vi "Example_SOM.vi"() -> ()   [LabVIEW 2009]
uses:
  <vilib>/addons/Machine Learning/Unsupervised Learning/ml_SOM_structure.ctl
  <vilib>/addons/Machine Learning/Unsupervised Learning/ml_SOM_Kohonen Para.ctl
  <vilib>/Utility/miscctls.llb/LV3DPointTypeDef.ctl
  <vilib>/addons/Machine Learning/Visualization/Plot SOM (3D).vi
  <vilib>/addons/Machine Learning/Utilities/Riffle (matrix).vi
  <vilib>/addons/Machine Learning/NILabs_MLT.lvlib
panel:
  in  "Data set":T1(ring)
  in  "Stopping criteria":cluster{"tolarence":dbl, "max iterations":i32}={"tolarence"=1e-05, "max iterations"=50}
  in  "Parameters":T2={"d0"=5.0, "k_d"=5000.0, "miu0"=0.5, "k_miu"=500.0}
  in  "Lattice structure":T3={"row"=7, "col"=7, "lattice type"=enum."rectangular"}
  in  "# of samples":i32=1024
  out "SOM in the data space":refnum<vi>(3d-picture)
  # "Introduction:\nSelf-Organizing Map (SOM) is used to learn four data sets which have different structures."
  # "Data samples (red dots)\nNeurons (green dots) are conneted according to SOM lattice structure."
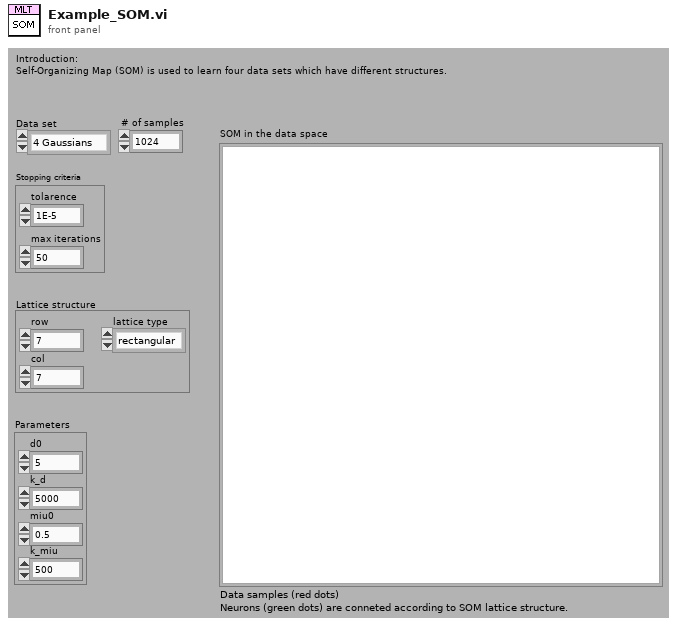
[diagram p1: front panel]
types:
  T1 = enum16{"4 Gaussians ", "uniform", "3 balls", "hemisphere"}
  T2 = typedef "NILabs_MLT.lvlib/ml_SOM_Kohonen Para.ctl" = cluster{"d0":dbl, "k_d":dbl, "miu0":dbl, "k_miu":dbl}
  T3 = typedef "NILabs_MLT.lvlib/ml_SOM_structure.ctl" = cluster{"row":i32, "col":i32, "lattice type":enum16{"rectangular", "hexagonal"}}
  T4 = typedef "LV3DPointTypeDef.ctl" = cluster{"X":sgl, "Y":sgl, "Z":sgl}
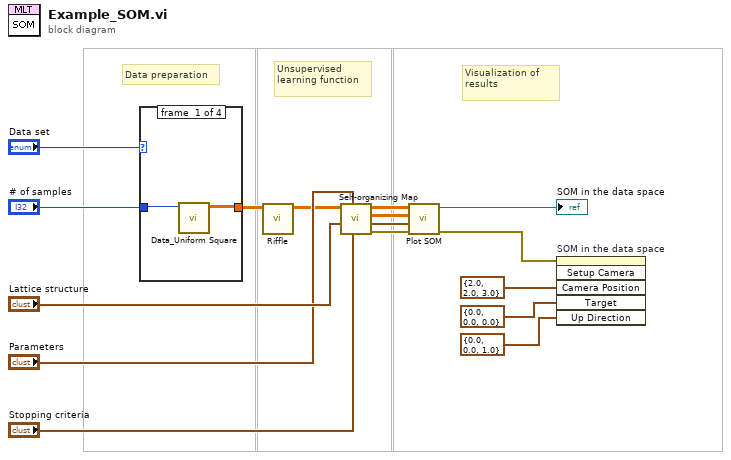
[diagram p0: block diagram]
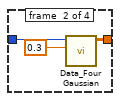
[diagram p2: hidden frame]
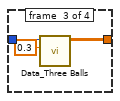
[diagram p3: hidden frame]
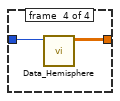
[diagram p4: hidden frame]
diagram:
  # "Visualization of results"
  # "Unsupervised learning function"
  # "Data preparation"
  n1 = case shown="\"3 balls\"" "Data set" {
    tunnel: "# of samples" -> [w18 w20 w23 w26]
    tunnel: [w17 w19 w24 w25] -> w2
    frame #0 {
      n2 = call "Data_Uniform Square.vi"("# of points"=w18) -> ("Data"=w17:dbl[][])  [unwired: 9 in, 1 out]
    }
    frame #1 {
      n3 = call "Data_Four Gaussian.vi"("noise amplitude"=0.3, "# of points"=w20) -> ("Data"=w19:dbl[][])  [unwired: 8 in, 1 out]
    }
    frame #2 {
      n4 = call "Data_Three Balls.vi"("noise amplitude"=0.3, "# of points"=w23) -> ("Data"=w24:dbl[][])  [unwired: 8 in, 1 out]
    }
    frame #3 {
      n5 = call "Data_Hemisphere.vi"("# of samples"=w26) -> ("Data samples"=w25:dbl[][])  [unwired: 9 in, 1 out]
    }
  }
  n6 = call-poly <vilib>:"Riffle.vi"("Data"=w2) -> ("Riffled{Data}"=w8:dbl[][])  [unwired: 8 in, 2 out]
  n7 = call <vilib>:"Self-organizing Map.vi"("stopping criteria"="Stopping criteria", "parameters"="Parameters", "lattice structure"="Lattice structure", "Data samples"=w8) -> ("error out"=w10:errorcluster, "structure dup"=w4:T3, "W"=w7:dbl[][], "Data samples dup"=w6:dbl[][])  [unwired: 4 in]
  n8 = call-poly <vilib>:"Plot SOM.vi"("error in (no error)"=w10, "structure"=w4, "W"=w7, "Data samples"=w6) -> ("error out"=w11:errorcluster, "3D Picture"=→"SOM in the data space":refnum<vi>)  [unwired: 6 in]
  n9 = invoke on="SOM in the data space" class="SceneGraphDisp (strict)" method="Setup Camera"(error in=w11, "Camera Position"=T4 {"X"=2.0, "Y"=2.0, "Z"=3.0}, "Target"=T4 {"X"=0.0, "Y"=0.0, "Z"=0.0} ("Camera Position"), "Up Direction"=T4 {"X"=0.0, "Y"=0.0, "Z"=1.0} ("Camera Position")) -> ()  [unwired: 2 in, 6 out]
